vi "vs digital filter3.vi"(4 "filter period(uSec)":i32, 5 "vs threshold":fxp<+/-,16,5>, 6 "input":dbl) -> (2 "output":bool)   [LabVIEW 2013]
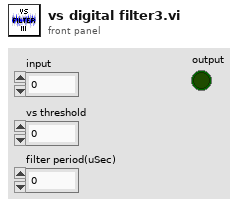
[diagram p1: front panel]
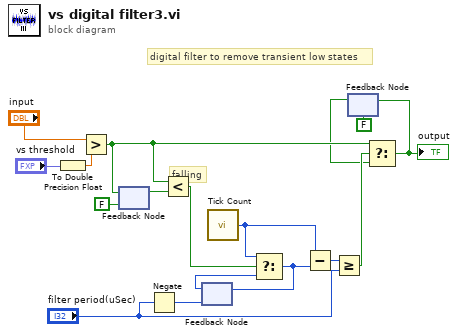
[diagram p0: block diagram]
diagram:
  # "digital filter to remove transient low states"
  # "falling"
  n1 = To Double Precision Float(number="vs threshold") -> (double precision float=w1:dbl)
  n2 = Greater?(x="input", y=w1) -> (0:w12:bool)
  n3 = feedback #1(FALSE) -> (w11:bool)
  n4 = feedback-in #1(w12) -> ()
  n5 = Negate(x="filter period(uSec)") -> (-x=w6:i32)
  n6 = Less?(x=w12, y=w11) -> (x < y?=w17:bool)
  n7 = feedback #2(w6) -> (w8:u32)
  n8 = call "Tick Count"() -> ("Tick Count(uSec)"=w16:u32)
  n9 = Select(t=w16, s=w17, f=w8) -> (s? t:f=w9:u32)
  n10 = feedback-in #2(w9) -> ()
  n11 = Subtract(x=w16, y=w9) -> (x-y=w15:u32)
  n12 = Greater Or Equal?(x=w15, y="filter period(uSec)") -> (x >= y?=w14:bool)
  n13 = feedback #3(FALSE) -> (w4:bool)
  n14 = Select(t=w12, s=w14, f=w4) -> (s? t:f=w5:bool)
  "output" <- w5
  n15 = feedback-in #3(w5) -> ()
